vi "Write OCP_Mode.vi"(8 "error in":errorcluster, 10 "OCP Mode":T1, 11 "6032A in":refnum<class "6032A.lvclass">) -> (0 "error out":errorcluster, 3 "6032A out":refnum<class "6032A.lvclass">)   [LabVIEW 2019, in "6032A.lvlib" / "6032A.lvclass"]
uses:
  Library/6032A.lvclass
  builds/Instruments/PowerSupply.lvlibp/Custom Controls/OCP Mode.ctl
  Library/6032A.lvclass/6032A.ctl
  builds/Instruments/PowerSupply.lvlibp/Library/PowerSupply.lvclass
  <instrlib>/Agilent 6XXX Series/Agilent 6XXX Series.lvlib
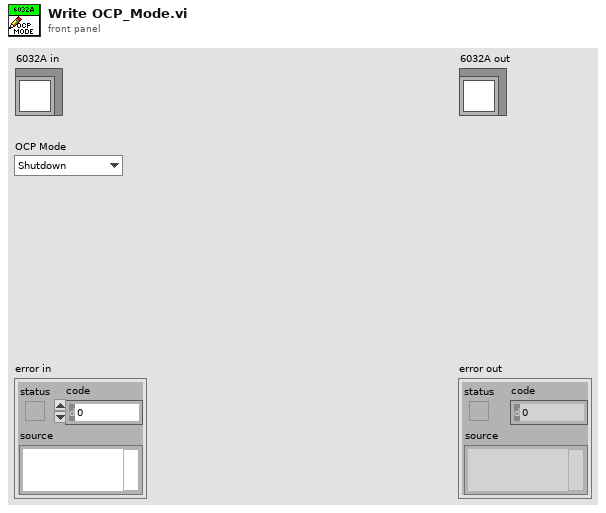
[diagram p1: front panel]
types:
  T1 = typedef "PowerSupply.lvlibp/PowerSupply.lvclass/OCP Mode.ctl" = enum16{"Shutdown", "Foldback"}
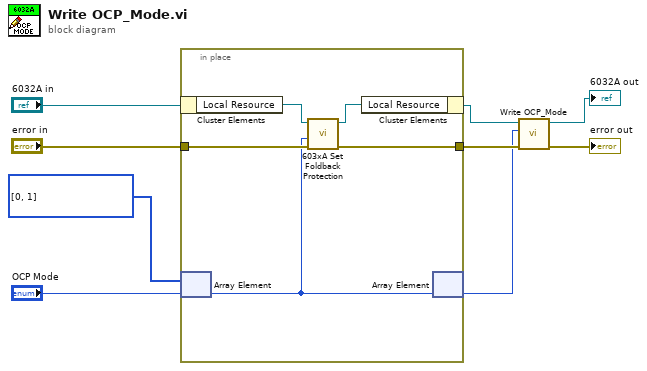
[diagram p0: block diagram]
diagram:
  w3 = u32[] [0, 1] items=["off", "constant voltage", "constant current"]
  n1 = in-place {
    in-place-border: "error in" -> [w12]
    in-place-border: [w11] -> w4
    n2 = in-place-cluster #1("6032A in") -> ("Local Resource"=w14:refnum<visa-resource-name>)
    n3 = in-place-array #2(w3, "OCP Mode") -> (w10:u32)
    n4 = call <instrlib>:"603xA Set Foldback Protection.vi"("error in (no error)"=w12, "foldback protection (0:off)"=w10, "VISA resource name"=w14) -> ("error out"=w11:errorcluster, "VISA resource name out"=w13:refnum<visa-resource-name>)  [unwired: 7 in]
    n5 = in-place-cluster #1("Local Resource"=w13) -> (w6:refnum<class "6032A.lvclass">)
    n6 = in-place-array #2(w10) -> (w1:i32)  [unwired: 1 out]
  }
  n7 = call-parent "Write OCP_Mode.vi"("error in"=w4, "OCP Mode"=w1, "PowerSupply in"=w6) -> ("error out"=→"error out":errorcluster, "PowerSupply out"=→"6032A out":refnum<class "6032A.lvclass">)  [unwired: 7 in]
